vi "VPI Init PWM.vi"(8 "error in (no error)":errorcluster, 9 "pInitConfig":T1, 10 "DevIndex":i32, 11 "DevType":i32) -> (0 "error out":errorcluster, 3 "function return":i32)   [LabVIEW 2012, in "ControlPWM.lvlib"]
doc: "int WINAPI VPI_InitPWM(int DevType, int DevIndex, PVPI_INIT_CONFIG pInitConfig);"
uses:
  ControlPWM.lvlib
  Ginkgo_Driver.dll
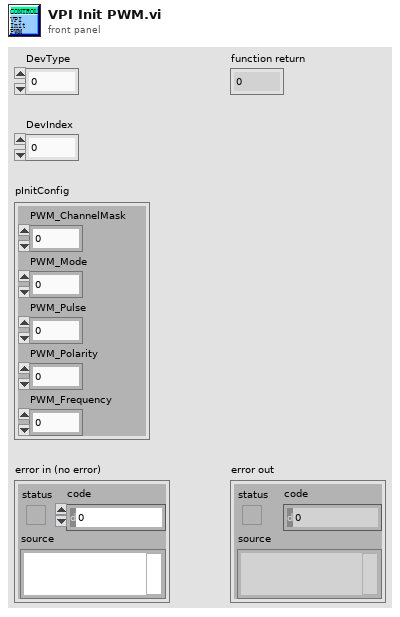
[diagram p1: front panel]
types:
  T1 = cluster{"PWM_ChannelMask":u8, "PWM_Mode":u8, "PWM_Pulse":u8, "PWM_Polarity":u8, "PWM_Frequency":u32}
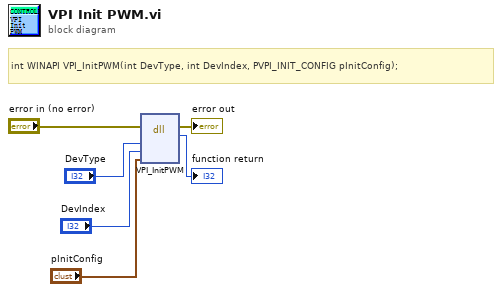
[diagram p0: block diagram]
diagram:
  # "int WINAPI VPI_InitPWM(int DevType, int DevIndex, PVPI_INIT_CONFIG pInitConfig);"
  n1 = dll-call lib="E:/Project/vt_ginkgo/truck/Ginkgo Driver/vs2010/Ginkgo_USB-I2C_API_v2.0.3.0/lib/labview_64bit/ControlPWM/Ginkgo_Driver.*" fn="VPI_InitPWM"(error in="error in (no error)", "DevType"="DevType", "DevIndex"="DevIndex", "pInitConfig"="pInitConfig") -> (error out=→"error out":errorcluster, →"function return":i32)  [unwired: 5 in, 1 out]
